vi "Determine Warnings.vi"() -> ()   [LabVIEW 2014]
panel:
  in  "Minimum Tempature":dbl
  in  "Maximum Tempature":dbl
  in  "Current Temp":dbl
  out "Warning Text":string
  out "Warning":bool
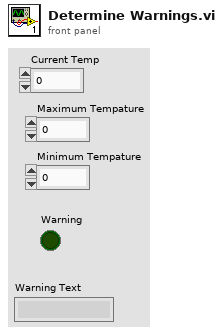
[diagram p1: front panel]
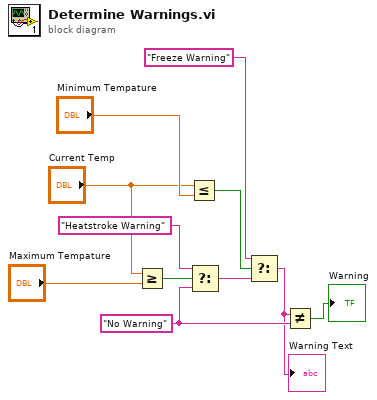
[diagram p0: block diagram]
diagram:
  w6 = "No Warning"
  n1 = Greater Or Equal?(x="Current Temp", y="Maximum Tempature") -> (x >= y?=w8:bool)
  n2 = Less Or Equal?(x="Current Temp", y="Minimum Tempature") -> (x <= y?=w5:bool)
  n3 = Select(t="Heatstroke Warning", s=w8, f=w6) -> (s? t:f=w3:string)
  n4 = Select(t="Freeze Warning", s=w5, f=w3) -> (s? t:f=w1:string)
  "Warning Text" <- w1
  n5 = Not Equal?(x=w1, y=w6) -> (x != y?=→"Warning":bool)
